vi "button_response.vi"(7 "LabVIEW Web Service Request":refnum<class "Web Request.lvclass">) -> ()   [LabVIEW 2015]
uses:
  <vilib>/wsapi/Web Request.lvclass
  global_cms.vi
panel:
  out "x = y?":bool
  # "Use the Web Service Request input terminal to call the VIs on the Web Services palette. Do not remove it from the connector pane unless you don't need access to the palette."
  # "Each additional control wired to the connector pane will be available as an input in the URL. To include an indicator in terminal-mode output (the default setting), it must also be wired to the connector pane."
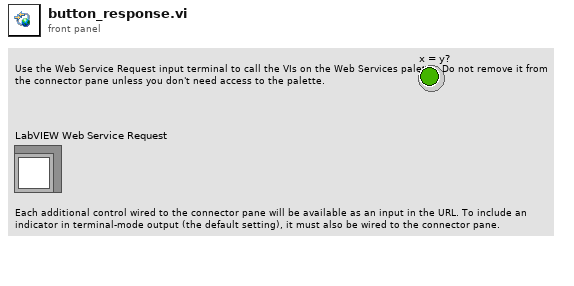
[diagram p1: front panel]
types:
  T1 = cluster{"_status":string, "_token":string, "result":string, "filePath":string}
  T2 = cluster{"data":cluster{"fileRequest":cluster{"filePath":string, "fileType":string, "fileName":string, "time":u32, "filePathTmp":string, "fileSize":u32}, "fileResponse":cluster{"filePath":string, "fileType":string, "fileName":string, "decode":string, "result":string, "status":string, "time":u32, "size":u32}}[], "_status":string, "_token":string}
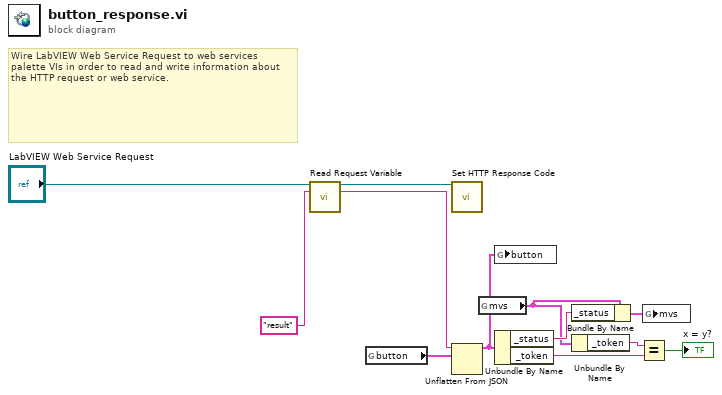
[diagram p0: block diagram]
diagram:
  # "Wire LabVIEW Web Service Request to web services palette VIs in order to read and write information about the HTTP request or web service."
  n1 = call <vilib>:"Read Request Variable.vi"("LabVIEW Web Service Request"="LabVIEW Web Service Request", "variable name"="result" ("key")) -> ("LabVIEW Web Service Request out"=w9:refnum<class "Web Request.lvclass">, "value"=w8:string)  [unwired: 11 in, 1 out]
  n2 = global read "global_cms.vi" "button"() -> (w12:T1)
  n3 = call <vilib>:"Set HTTP Response Code.vi"("LabVIEW Web Service Request"=w9) -> ()  [unwired: 13 in, 2 out]
  n4 = Unflatten From JSON(JSON string=w8, type and defaults=w12) -> (value=w6:T1)  [unwired: 5 in, 1 out]
  n5 = global read "global_cms.vi" "mvs"() -> (w3:T2)
  n6 = global write "global_cms.vi" "button"(w6) -> ()
  n7 = Unbundle By Name(w6) -> ("_status"=w5:string, "_token"=w4:string)
  n8 = Bundle By Name(cluster=w3, "_status"=w5) -> (w7:T2)
  n9 = Unbundle By Name(w3) -> ("_token"=w2:string)
  n10 = Equal?(x=w2, y=w4) -> (x = y?=→"x = y?":bool)
  n11 = global write "global_cms.vi" "mvs"(w7) -> ()
